vi "Cieślikiewicz_0.vi"() -> ()   [LabVIEW 2020]
panel:
  out "Numeric":dbl
  in  "stop":bool
  in  "Boolean 3":bool
  in  "Boolean 2":bool
  in  "Boolean":bool
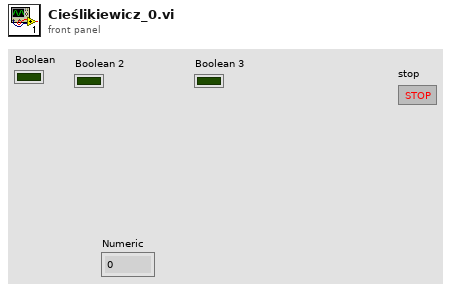
[diagram p1: front panel]
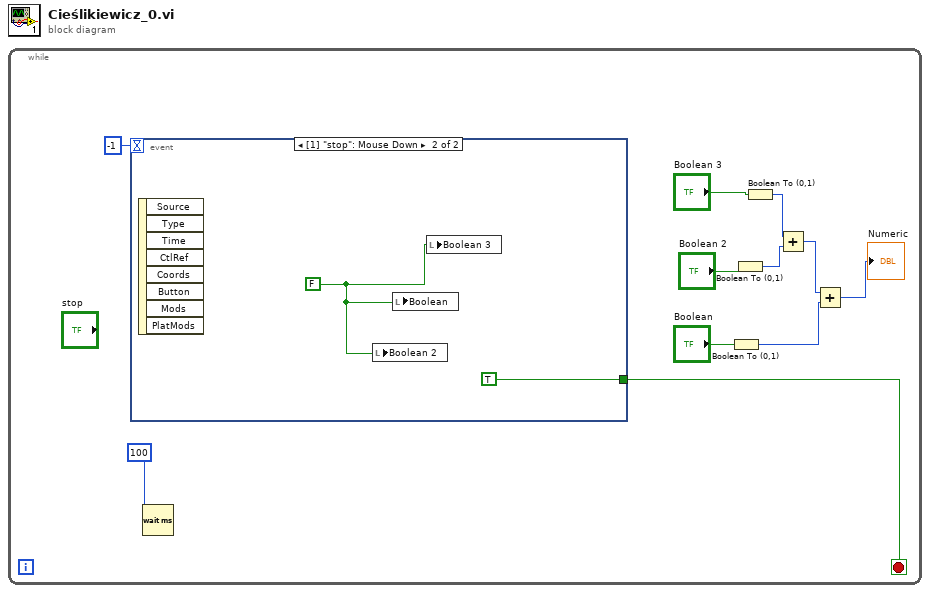
[diagram p0: block diagram]
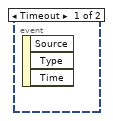
[diagram p2: hidden frame]
diagram:
  n1 = while {
    stop <- w9 stop-if-true
    n2 = event shown="[1] \"stop\": Mouse Down" {
      selector: _ -> [_ _]
      dyn-events: _ -> [_ _]
      timeout: -1 -> [_ _]
      tunnel: [_ TRUE] -> w9
      event Timeout {
        n3 = event-data() -> ()  [unwired: 1 in, 3 out]
      }
      event "stop": Mouse Down {
        w13 = FALSE
        n4 = event-data() -> ()  [unwired: 1 in, 8 out]
        n5 = local write "Boolean 2"(w13) -> ()
        n6 = local write "Boolean"(w13) -> ()
        n7 = local write "Boolean 3"(w13) -> ()
      }
    }
    n8 = Wait (ms)(milliseconds to wait=u32 100) -> ()  [unwired: 1 out]
    n9 = Boolean To (0,1)(Boolean="Boolean") -> (0, 1=w2:i16)
    n10 = Boolean To (0,1)(Boolean="Boolean 2") -> (0, 1=w4:i16)
    n11 = Boolean To (0,1)(Boolean="Boolean 3") -> (0, 1=w5:i16)
    n12 = Add(x=w5, y=w4) -> (x+y=w3:i16)
    n13 = Add(x=w3, y=w2) -> (x+y=→"Numeric":i16)
  }
